vi "BRig_Host__Loop_Producer__tcp_System__Data_checkExistence_arrFilepath.vi"(8 "input_I_arrPath":bool[](array[boolean]), 9 "input_n":i32, 11 "input_arrPath":path[](array[path])) -> (3 "output_exist":bool[](array[boolean]))   [LabVIEW 2014]
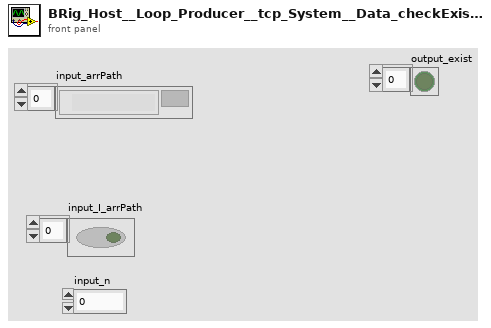
[diagram p1: front panel]
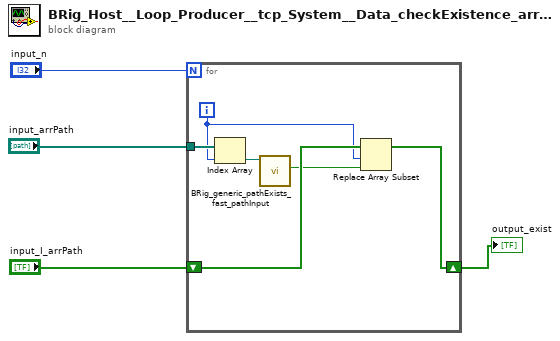
[diagram p0: block diagram]
diagram:
  n1 = for {
    N: "input_n" -> [_]
    tunnel: "input_arrPath" -> [w10]
    shift-right: [w7] -> w1
    shift-left: "input_I_arrPath" -> [w9]
    i -> [w8]
    n2 = Index Array(array=w10, index=w8) -> (element=w6:path)
    n3 = call "BRig_generic_pathExists_fast_pathInput.vi"("input_filePath"=w6) -> ("output_Iexist"=w5:bool)  [unwired: 8 in, 2 out]
    n4 = Replace Array Subset(array=w9, new element=w5, index=w8) -> (w7:bool[])
  }
  "output_exist" <- w1
